vi "WriteButtonBar.vi"(8 "Error In":errorcluster, 10 "ButtonBar":refnum<class "ButtonCollection.lvclass"> caption="Object Out", 11 "reference in":refnum<class "VerticalButtonBar.lvclass">) -> (0 "Error Out":errorcluster, 3 "reference in":refnum<class "VerticalButtonBar.lvclass">)   [LabVIEW 2021, in "VerticalButtonBar.lvclass"]
uses:
  VerticalButtonBar.lvclass
  ButtonCollection/ButtonCollection.lvclass
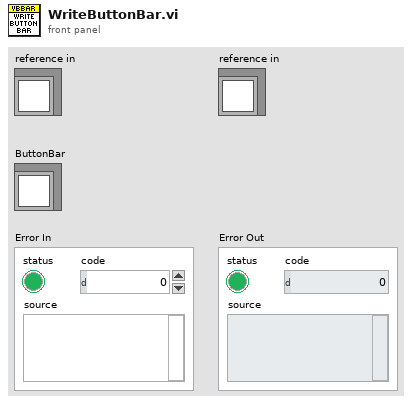
[diagram p1: front panel]
types:
  T1 = typedef "VerticalButtonBar.lvclass/ObjectAttributes.ctl" = cluster{"Interfaces":cluster{"IDockGUI":refnum<class "IDockGUI.lvclass">, "Authorizer":refnum<class "IAuthorization.lvclass">}, "Locals":cluster{"ButtonBar":refnum<class "ButtonCollection.lvclass">, "BaseConfigurationPath":path, "Labels":cluster{"Label":string, "Value":string}[]}, "Persistent":cluster{"ButtonDefinitionFile":string}}
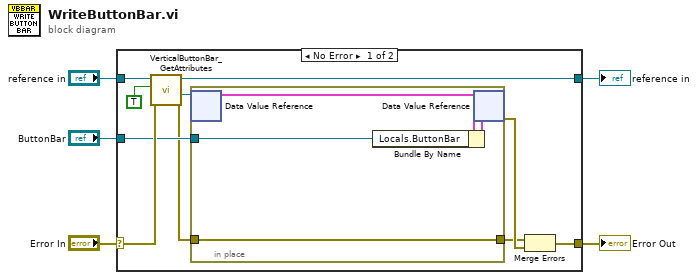
[diagram p0: block diagram]
diagram:
  n1 = case shown="No Error" "Error In" {
    selector: "Error In" -> [w13 w21]
    tunnel: [w9 w21] -> w4
    tunnel: [w14 w20] -> w2
    tunnel: "reference in" -> [w15 w20]
    tunnel: "ButtonBar" -> [w8 _]
    frame No Error {
      n2 = call "VerticalButtonBar_GetAttributes.vi"("error in (no error)"=w13, "OnlyGetDvrReference(False)"=TRUE, "reference in"=w15) -> ("error out"=w7:errorcluster, "DataRef"=w10:refnum<data-value>, "reference out"=w14:refnum<class "VerticalButtonBar.lvclass">)  [unwired: 5 in, 1 out]
      n3 = in-place {
        in-place-border: w8 -> [w16]
        in-place-border: w7 -> [w17]
        in-place-border: [w17] -> w6
        n4 = in-place-dvr #1(w10) -> (w18:T1)  [unwired: 1 out]
        n5 = Bundle By Name(cluster=w18, "Locals.ButtonBar"=w16) -> (w19:T1)
        n6 = in-place-dvr #1(w19) -> (w11:errorcluster)  [unwired: 1 out]
      }
      n7 = Merge Errors(w6, w11) -> (w9:errorcluster)
    }
    frame Error {
    }
  }
  "Error Out" <- w4
  "reference in" <- w2
